vi "Set Configuration.vi"(8 "error in (no error)":errorcluster, 11 "Digital Static Input in":refnum<class "Digital Static Input.lvclass">) -> (0 "error out":errorcluster, 3 "Digital Static Input out":refnum<class "Digital Static Input.lvclass">)   [LabVIEW 2015, in "Digital Static Input.lvclass"]
uses:
  Digital Static Input.lvclass
  IO Class/Type.ctl
  FPGA Addon Input/FPGA Addon Input.lvclass
  IO Class/IO Class.lvclass
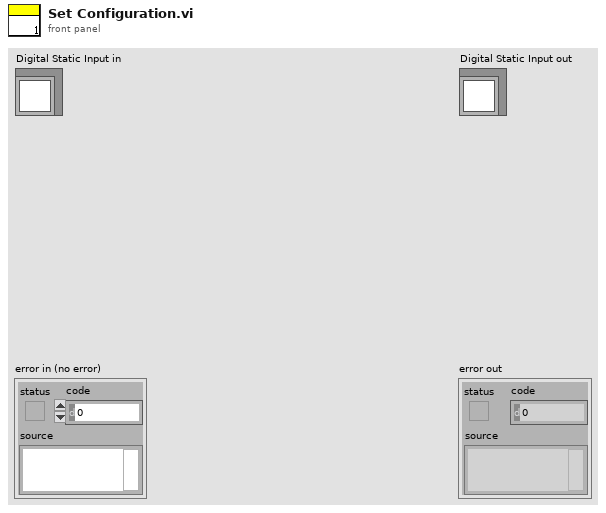
[diagram p1: front panel]
types:
  T1 = typedef "IO Class.lvclass/Type.ctl" = cluster{"Type":string}
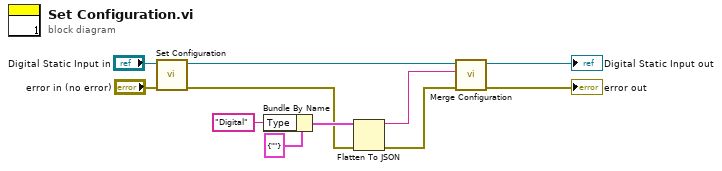
[diagram p0: block diagram]
diagram:
  n1 = call-parent "Set Configuration.vi"("error in (no error)"="error in (no error)", "FPGA Addon Input in"="Digital Static Input in") -> ("error out"=w2:errorcluster, "FPGA Addon Input out"=w4:refnum<class "Digital Static Input.lvclass">)  [unwired: 8 in]
  n2 = Bundle By Name(cluster=T1 {"Type"=""} ("Type"), "Type"="Digital") -> (w8:T1)
  n3 = Flatten To JSON(anything=w8, error in (no error)=w2) -> (JSON string=w7:string, 11:w6:errorcluster)  [unwired: 1 in]
  n4 = call "Merge Configuration.vi"("error in (no error)"=w6, "Additional Configuration"=w7, "IO Class in"=w4) -> ("error out"=→"error out":errorcluster, "IO Class out"=→"Digital Static Input out":refnum<class "Digital Static Input.lvclass">)  [unwired: 7 in]
